vi "Main.vi"(8 "error in":errorcluster, 11 "Settings Window in":refnum<class "Settings Window.lvclass">) -> (0 "error out":errorcluster, 3 "Settings Window out":refnum<class "Settings Window.lvclass">)   [LabVIEW 2023, in "Settings Window.lvclass"]
doc: "The <b>Queued Message Handler</b> of the Worker that owns this VI."
uses:
  Settings Window.lvclass
  Settings.ctl
  Initialization Data.ctl
  Response Cases.ctl
  <vilib>/addons/_Workers/Library/Case Label.ctl
  Settings Window.lvclass/Settings Window.ctl
  rqp_Show Window.ctl
  rqp_Get Settings.ctl
  <vilib>/Utility/error.llb/Error Cluster From Error Code.vi
  <vilib>/ErrorRing/Error Ring.xnode
  <vilib>/addons/_Workers/Library/Classes/Message Queue/Message Queue.lvclass
  <vilib>/addons/_Workers/Library/Workers.lvlib
panel:
  in  "Calcs":T1 caption="Расчёты" {"B" format="%#_f"; "b" format="%#_f"; "A" format="%#_f"; "a" format="%#_f"; "K0" format="%#_f"; "Vm0" format="%#_f"}
  in  "Read Calcs":bool
  in  "Cancel Button":bool
  in  "OK Button":bool
  in  "Read Heater":bool
  in  "Heater":cluster{"P":dbl, "I":dbl} caption="Нагреватель" {"I" format="%#_f"; "P" format="%#_f"}
  in  "Read PLC2":bool
  in  "Read PLC1":bool
  in  "PLC2":cluster{"port":u16, "address":string}
  in  "PLC1":cluster{"port":u16, "address":string}
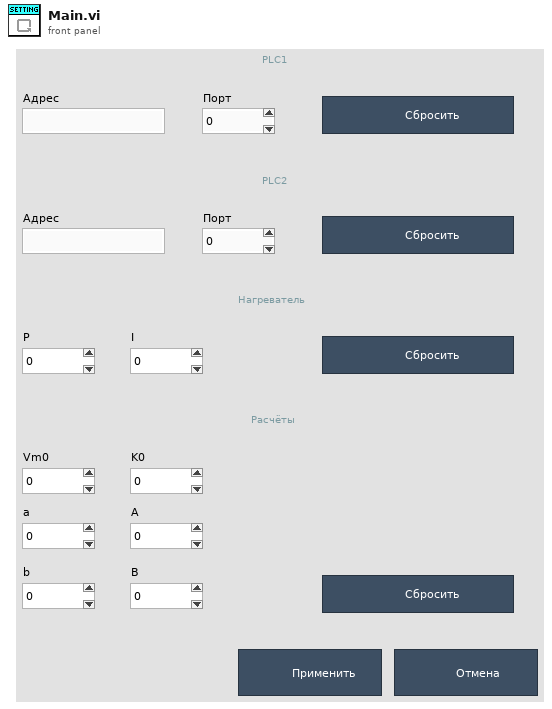
[diagram p1: front panel]
types:
  T1 = cluster{"Vm0":dbl, "K0":dbl, "a":dbl, "A":dbl, "b":dbl, "B":dbl}
  T2 = enum32{"Invalid", "Standard", "Closed", "Hidden", "Minimized", "Maximized"}
  T3 = typedef "Settings Window.lvclass/Settings.ctl" = cluster{"PLC1":cluster{"port":u16, "address":string}, "PLC2":cluster{"port":u16, "address":string}, "Heater":cluster{"P":dbl, "I":dbl}, "Calcs":cluster{"Vm0":dbl, "K0":dbl, "a_small":dbl, "A":dbl, "b_small":dbl, "B":dbl}}
  T4 = cluster{"PLC1":cluster{"port":u16, "address":string}, "PLC2":cluster{"port":u16, "address":string}, "Heater":cluster{"P":dbl, "I":dbl}, "Calcs":cluster{"Vm0":dbl, "K0":dbl, "a_small":dbl, "A":dbl, "b_small":dbl, "B":dbl}}
  T5 = typedef "Settings Window.lvclass/Initialization Data.ctl" = cluster{"Response Cases":T6, "Config Path":path}
  T6 = typedef "Settings Window.lvclass/Response Cases.ctl" = cluster{"Placeholder - Can be deleted":string, "Get Settings":T7, "Starting Settings":T7}
  T7 = typedef "Workers.lvlib/Case Label.ctl" = string
  T8 = enum16{"open", "replace", "create", "open or create", "replace or create", "replace or create with confirmation"}
  T9 = typedef "Settings Window.lvclass/rqp_Show Window.ctl" = cluster{"String":string}
  T10 = typedef "Settings Window.lvclass/rqp_Get Settings.ctl" = cluster{"String":string}
  T11 = cluster{"Vm0":dbl, "K0":dbl, "a_small":dbl, "A":dbl, "b_small":dbl, "B":dbl}
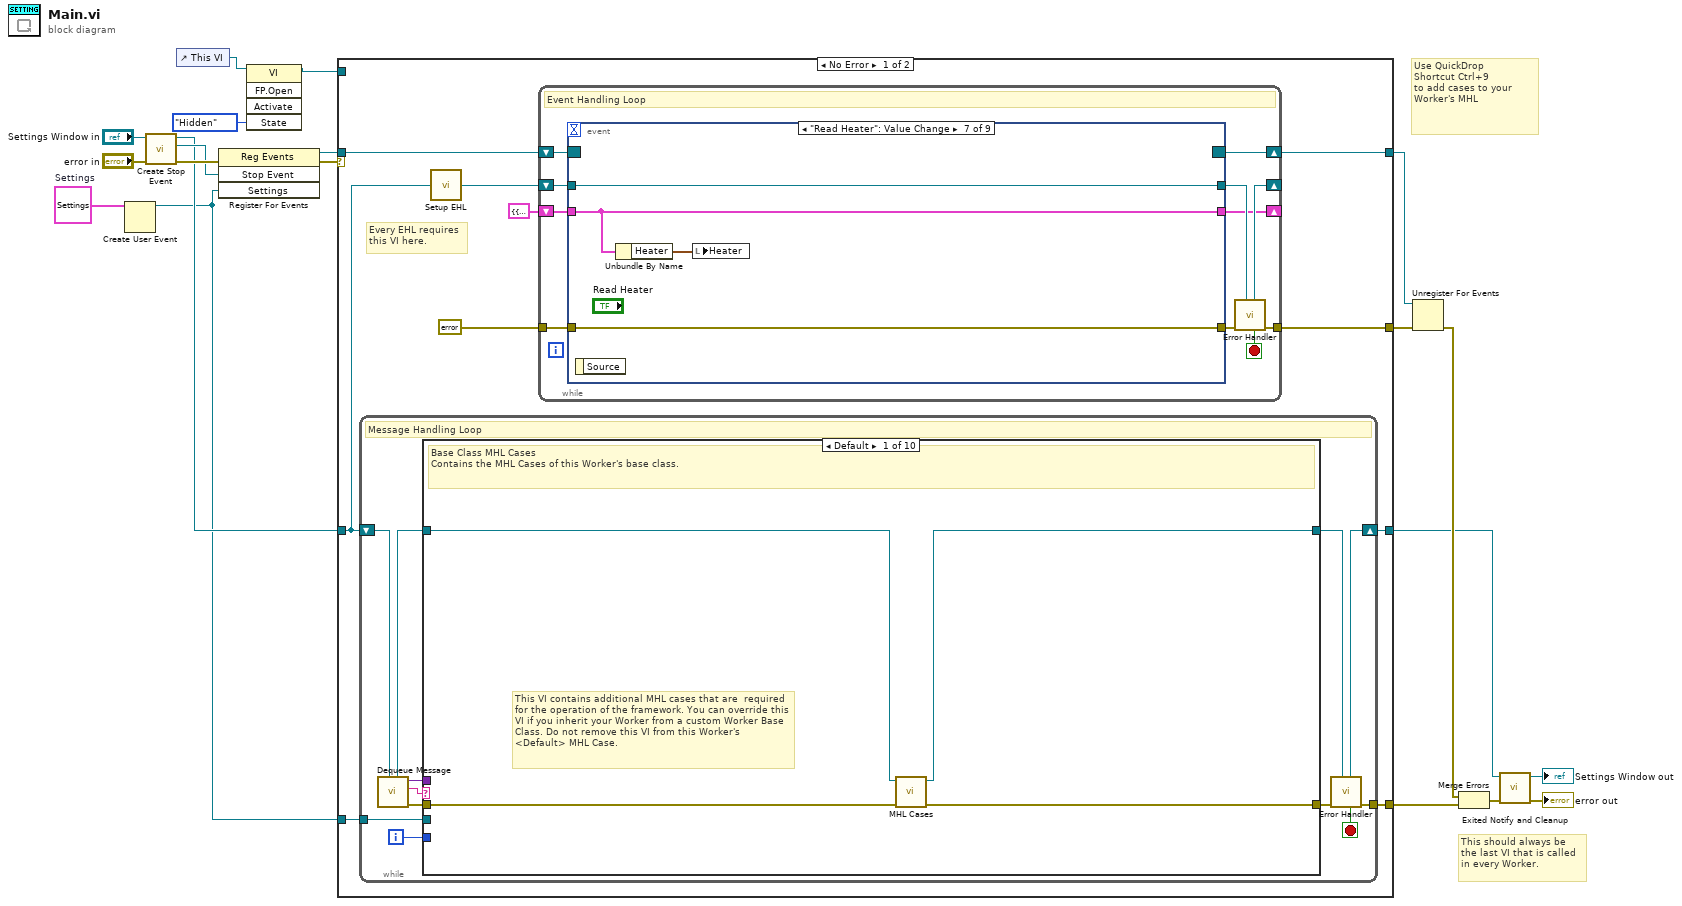
[diagram p0: block diagram]
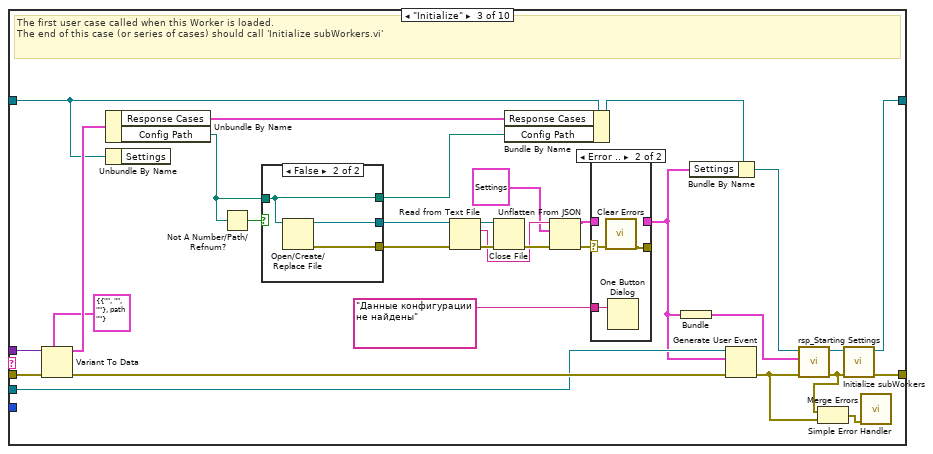
[diagram p3: hidden frame]
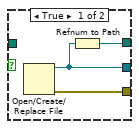
[diagram p5: hidden frame]
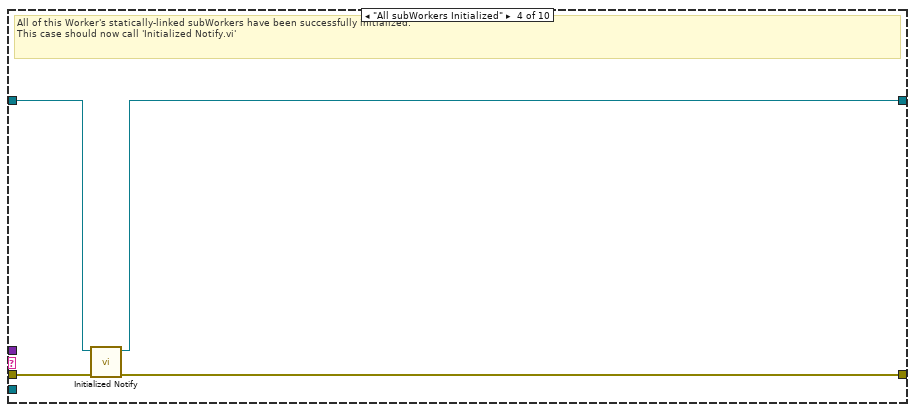
[diagram p6: hidden frame]
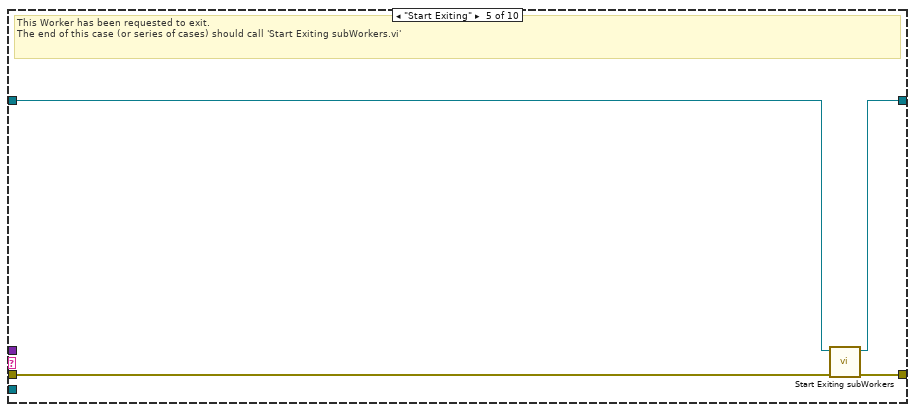
[diagram p7: hidden frame]
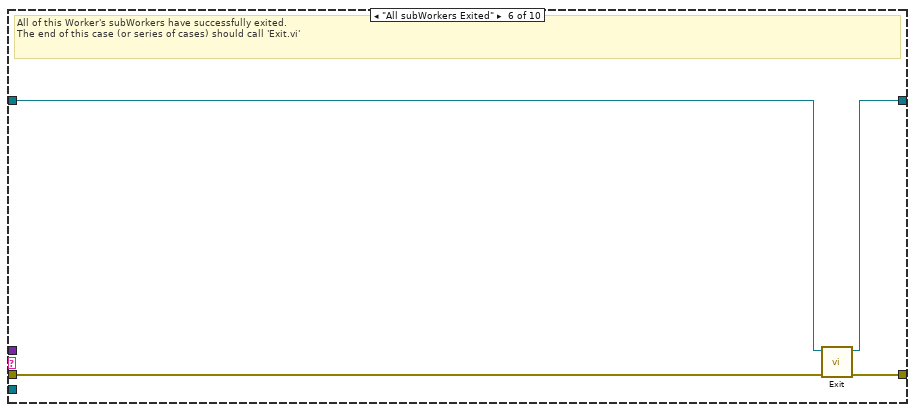
[diagram p8: hidden frame]
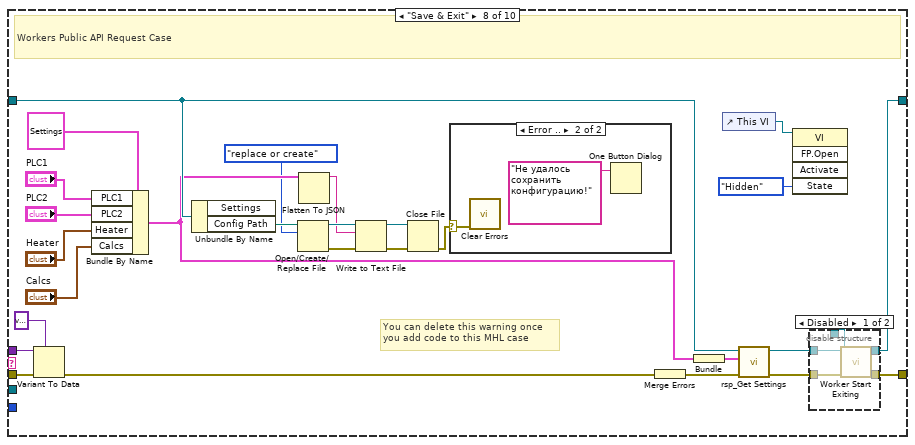
[diagram p10: hidden frame]
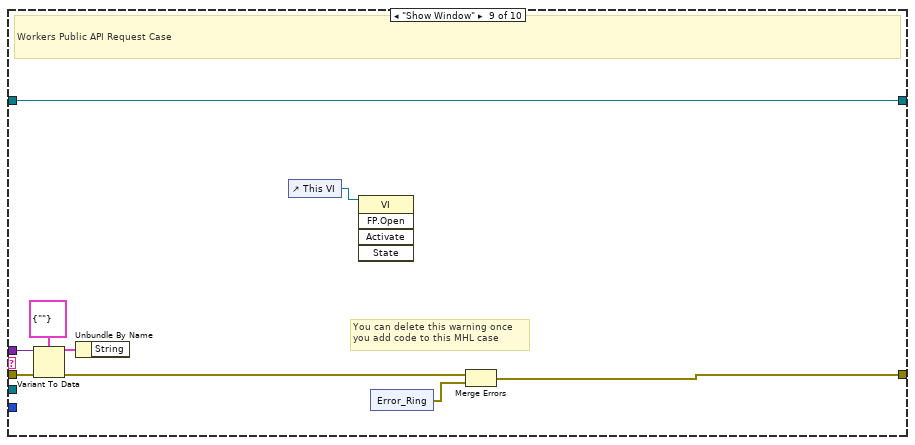
[diagram p13: hidden frame]
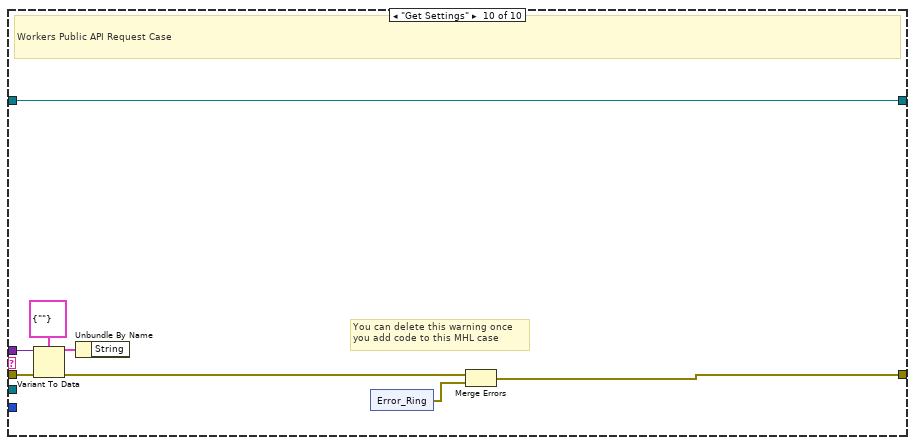
[diagram p14: hidden frame]
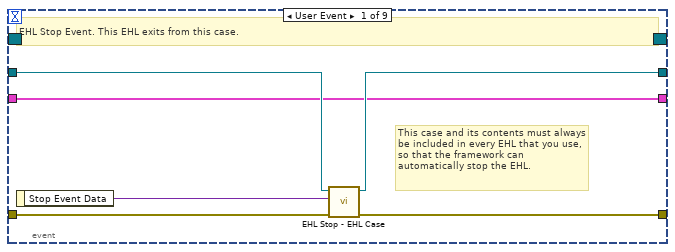
[diagram p15: hidden frame]
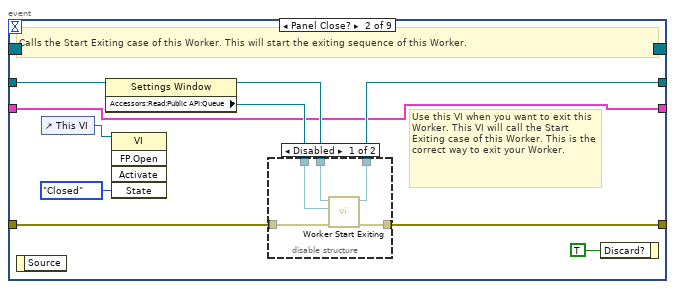
[diagram p16: hidden frame]
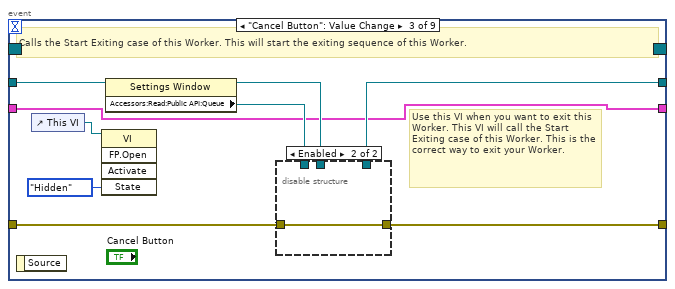
[diagram p18: hidden frame]
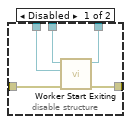
[diagram p19: hidden frame]
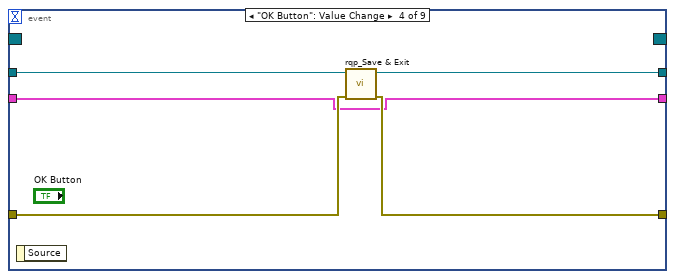
[diagram p20: hidden frame]
diagram:
  w4 = T3 {"PLC1"={"port"=0, "address"=""}, "PLC2"={"port"=0, "address"=""}, "Heater"={"P"=0.0, "I"=0.0}, "Calcs"={"Vm0"=0.0, "K0"=0.0, "a_small"=0.0, "A"=0.0, "b_small"=0.0, "B"=0.0}}  # Settings
  # "Use QuickDrop\nShortcut Ctrl+9\nto add cases to your\nWorker's MHL"
  # "This should always be the last VI that is called in every Worker."
  n1 = Create User Event(user event datatype=w4) -> (user event=w5:refnum<user-event>)  [unwired: 1 in, 1 out]
  n2 = call-dynamic "Create Stop Event.vi"("error in"="error in", "Worker"="Settings Window in") -> ("error out"=w15:errorcluster, "Stop Event"=w12:refnum<user-event>, "Worker out"=w9:refnum<class "Settings Window.lvclass">)  [unwired: 7 in]
  n3 = control-ref of="This VI"() -> (w3:refnum<vi>)
  n4 = register-events(error in=w15, w12, w5) -> (reference out=w14:refnum<event-registration>, error out=w6:errorcluster)  [unwired: 1 in]
  n5 = invoke class="VI" method="FP.Open"(reference=w3, "State"=T2."Hidden") -> (reference out=w1:refnum<vi>)  [unwired: 3 in, 4 out]
  n6 = case shown="No Error" w6 {
    tunnel: w9 -> [w22 w245]
    tunnel: [w24 w246] -> w13
    tunnel: w14 -> [w30 w247]
    tunnel: [w27 w248] -> w19
    tunnel: [w29 w247] -> w18
    tunnel: [w25 w244] -> w16
    selector: w6 -> [_ w248]
    tunnel: w5 -> [w23 _]
    tunnel: w1 -> [_ _]
    frame No Error {
      # "Every EHL requires\nthis VI here."
      n7 = while {
        shift-right: [w40] -> w25
        shift-left: w22 -> [w42]
        tunnel: [w41] -> w24
        tunnel: w23 -> [w32]
        i -> [w33]
        stop <- w34 stop-if-true
        # "Message Handling Loop"
        n8 = call-dynamic "Dequeue Message.vi"("Worker"=w42) -> ("error out"=w39:errorcluster, "Case out"=w35:string, "Data out"=w31:variant, "Worker out"=w37:refnum<class "Settings Window.lvclass">)  [unwired: 6 in, 1 out]
        n9 = case "Worker MHL Case Structure (DO NOT CHANGE LABEL NAME)" shown="Default" w35 {
          tunnel: w39 -> [w46 w47 w78 w92 w95 w102 w104 w131 w148 w161]
          tunnel: [w45 w47 w53 w91 w98 w101 w104 w117 w143 w156] -> w38
          tunnel: w37 -> [w44 w48 w68 w94 w96 w100 w103 w119 w149 w162]
          tunnel: [w43 w48 w79 w93 w97 w99 w103 w116 w149 w162] -> w36
          tunnel: w33 -> [_ _ _ _ _ _ _ _ _ _]
          tunnel: w32 -> [_ _ w61 _ _ _ _ _ _ _]
          tunnel: w31 -> [_ _ w77 _ _ _ _ w129 w145 w158]
          frame Default {
            # "This VI contains additional MHL cases that are  required for the operation of the framework. You can override this VI if you inherit your Worker from a custom Worker Base Class. Do not remove this VI from this Worker's <Default> MHL Case."
            # "Base Class MHL Cases\nContains the MHL Cases of this Worker's base class."
            n10 = call-dynamic "MHL Cases.vi"("error in"=w46, "Worker in"=w44) -> ("error out"=w45:errorcluster, "Worker out"=w43:refnum<class "Settings Window.lvclass">)  [unwired: 8 in]
          }
          frame "------------ FRAMEWORK CASES -----------" {
            # "Start of Workers Framework Cases"
          }
          frame "Initialize" {
            # "The first user case called when this Worker is loaded.\nThe end of this case (or series of cases) should call 'Initialize subWorkers.vi'"
            n11 = Variant To Data(error in=w78, type=T5 {"Response Cases"={"Placeholder - Can be deleted"="", "Get Settings"="", "Starting Settings"=""}, "Config Path"=path ""} ("Initialization Data"), Variant=w77) -> (data=w76:T5, error out=w62:errorcluster)
            n12 = Unbundle By Name(w76) -> ("Response Cases"=w75:T6, "Config Path"=w54:path)
            n13 = Unbundle By Name(w68) -> ()  [unwired: 1 out]
            n14 = Not A Number/Path/Refnum?(number/path/refnum=w54) -> (NaN/Path/Refnum?=w73:bool)
            n15 = case shown="False" w73 {
              tunnel: [w86 w90] -> w60
              tunnel: w54 -> [_ w88]
              tunnel: [w87 w89] -> w72
              tunnel: [w85 w88] -> w59
              frame True {
                n16 = Open/Create/Replace File() -> (refnum out=w86:refnum<file>, error out=w87:errorcluster)  [unwired: 6 in, 1 out]
                n17 = Refnum to Path(1:w86) -> (0:w85:path)
              }
              frame False {
                n18 = Open/Create/Replace File(file path (use dialog)=w88) -> (refnum out=w90:refnum<file>, error out=w89:errorcluster)  [unwired: 5 in, 1 out]
              }
            }
            n19 = Read from Text File(file (use dialog)=w60, error in=w72) -> (refnum out=w70:refnum<file>, text=w67:string, error out=w71:errorcluster)  [unwired: 2 in, 1 out]
            n20 = Close File(refnum=w70, error in=w71) -> (error out=w69:errorcluster)  [unwired: 1 out]
            n21 = Bundle By Name(cluster=w68, "Response Cases"=w75, "Config Path"=w59) -> (w63:refnum<class "Settings Window.lvclass">)
            n22 = Unflatten From JSON(JSON string=w67, type and defaults=T3 {"PLC1"={"port"=0, "address"=""}, "PLC2"={"port"=0, "address"=""}, "Heater"={"P"=0.0, "I"=0.0}, "Calcs"={"Vm0"=0.0, "K0"=0.0, "a_small"=0.0, "A"=0.0, "b_small"=0.0, "B"=0.0}} ("Settings"), error in (no error)=w69) -> (value=w65:T3, error out=w66:errorcluster)  [unwired: 4 in]
            n23 = case shown="Error .." w66 {
              selector: w66 -> [w80 w84]
              tunnel: [w81 _] -> w58
              tunnel: w65 -> [w81 _]
              tunnel: [w80 w83] -> _
              tunnel: "Данные конфигурации не найдены" ("message") -> [_ w82]
              frame No Error {
              }
              frame Error {
                n24 = call <vilib>:"Clear Errors.vi"("error in (no error)"=w84) -> ("error out"=w83:errorcluster)  [unwired: 5 in, 1 out]
                n25 = One Button Dialog(message=w82) -> ()  [unwired: 1 in, 1 out]
              }
            }
            n26 = Bundle("Settings"=w58) -> (w57:cluster{"Settings":T3})  [unwired: 1 in]
            n27 = Bundle By Name(cluster=w63, "Settings"=w58) -> (w56:refnum<class "Settings Window.lvclass">)
            n28 = Generate User Event(user event=w61, event data cluster=w58, error in=w62) -> (error out=w50:errorcluster)  [unwired: 1 in, 1 out]
            n29 = call "rsp_Starting Settings.vi"("error in"=w50, "Data in"=w57, "Settings Window in"=w56) -> ("error out"=w51:errorcluster, "dup Settings Window out"=w55:refnum<class "Settings Window.lvclass">)  [unwired: 7 in]
            n30 = Merge Errors(w51, w50) -> (w52:errorcluster)
            n31 = call-dynamic "Initialize subWorkers.vi"("error in"=w51, "Worker"=w55) -> ("error out"=w53:errorcluster, "dup Worker out"=w79:refnum<class "Settings Window.lvclass">)  [unwired: 8 in]
            n32 = call <vilib>:"Simple Error Handler.vi"("error in (no error)"=w52) -> ()  [unwired: 4 in, 5 out]
          }
          frame "All subWorkers Initialized" {
            # "All of this Worker's statically-linked subWorkers have been successfully initialized.\nThis case should now call 'Initialized Notify.vi'"
            n33 = call-dynamic "Initialized Notify.vi"("error in"=w92, "Worker"=w94) -> ("error out"=w91:errorcluster, "dup Worker out"=w93:refnum<class "Settings Window.lvclass">)  [unwired: 8 in]
          }
          frame "Start Exiting" {
            # "This Worker has been requested to exit. \nThe end of this case (or series of cases) should call 'Start Exiting subWorkers.vi'"
            n34 = call-dynamic "Start Exiting subWorkers.vi"("error_in"=w95, "Worker"=w96) -> ("error out"=w98:errorcluster, "dup Worker out"=w97:refnum<class "Settings Window.lvclass">)  [unwired: 8 in]
          }
          frame "All subWorkers Exited" {
            # "All of this Worker's subWorkers have successfully exited. \nThe end of this case (or series of cases) should call 'Exit.vi'"
            n35 = call-dynamic "Exit.vi"("error_in"=w102, "Worker"=w100) -> ("error out"=w101:errorcluster, "dup Worker out"=w99:refnum<class "Settings Window.lvclass">)  [unwired: 8 in]
          }
          frame "------------- PUBLIC API CASES -------------" {
            # "Start of Workers Public API Cases"
          }
          frame "Save & Exit" {
            # "You can delete this warning once\nyou add code to this MHL case"
            # "Workers Public API Request Case"
            n36 = Variant To Data(error in=w131, type=variant, Variant=w129) -> (error out=w130:errorcluster)  [unwired: 1 out]
            n37 = Bundle By Name(cluster=T3 {"PLC1"={"port"=0, "address"=""}, "PLC2"={"port"=0, "address"=""}, "Heater"={"P"=0.0, "I"=0.0}, "Calcs"={"Vm0"=0.0, "K0"=0.0, "a_small"=0.0, "A"=0.0, "b_small"=0.0, "B"=0.0}} ("Settings"), "PLC1"="PLC1", "PLC2"="PLC2", "Heater"="Heater", "Calcs"="Calcs") -> (w111:T3)
            n38 = Unbundle By Name(w119) -> ("Config Path"=w128:path)  [unwired: 1 out]
            n39 = Open/Create/Replace File(file path (use dialog)=w128, operation (0:open)=T8."replace or create") -> (refnum out=w126:refnum<file>, error out=w127:errorcluster)  [unwired: 4 in, 1 out]
            n40 = Flatten To JSON(anything=w111) -> (JSON string=w122:string)  [unwired: 2 in, 1 out]
            n41 = Write to Text File(file (use dialog)=w126, text=w122, error in=w127) -> (refnum out=w120:refnum<file>, error out=w121:errorcluster)  [unwired: 1 in, 1 out]
            n42 = Close File(refnum=w120, error in=w121) -> (error out=w114:errorcluster)  [unwired: 1 out]
            n43 = case shown="Error .." w114 {
              selector: w114 -> [_ w139]
              frame No Error {
              }
              frame Error {
                n44 = call <vilib>:"Clear Errors.vi"("error in (no error)"=w139) -> ()  [unwired: 5 in, 2 out]
                n45 = One Button Dialog(message="Не удалось сохранить конфигурацию!") -> ()  [unwired: 1 in, 1 out]
              }
            }
            n46 = Merge Errors(w130) -> (w118:errorcluster)
            n47 = Bundle("Settings"=w111) -> (w109:cluster{"Settings":T3})  [unwired: 1 in]
            n48 = control-ref of="This VI"() -> (w107:refnum<vi>)
            n49 = call "rsp_Get Settings.vi"("error in"=w118, "Data in"=w109, "Settings Window in"=w119) -> ("error out"=w112:errorcluster, "dup Settings Window out"=w113:refnum<class "Settings Window.lvclass">)  [unwired: 7 in]
            n50 = invoke class="VI" method="FP.Open"(reference=w107, "State"=T2."Hidden") -> ()  [unwired: 3 in, 5 out]
            n51 = disable-structure shown="Disabled" {
              disable-tunnel: [w136 w137] -> w117
              disable-tunnel: _ -> [w135 _]
              disable-tunnel: [w134 w138] -> w116
              disable-tunnel: w113 -> [w133 w138]
              disable-tunnel: w112 -> [w132 w137]
              frame Disabled {
                n52 = call-dynamic "Worker Start Exiting.vi"("error_in"=w132, "Message Queue"=w135, "Worker"=w133) -> ("error out"=w136:errorcluster, "dup Worker out"=w134:refnum<class "Settings Window.lvclass">)  [unwired: 7 in]
              }
              frame Enabled {
              }
            }
          }
          frame "Show Window" {
            # "You can delete this warning once\nyou add code to this MHL case"
            # "Workers Public API Request Case"
            n53 = Variant To Data(error in=w148, type=T9 {"String"=""} ("Data"), Variant=w145) -> (data=w144:T9, error out=w147:errorcluster)
            n54 = Unbundle By Name(w144) -> ()  [unwired: 1 out]
            n55 = control-ref of="This VI"() -> (w141:refnum<vi>)
            n56 = invoke class="VI" method="FP.Open"(reference=w141) -> ()  [unwired: 4 in, 5 out]
            n57 = xnode ("Error_Ring")() -> ("error out"=w142:errorcluster)
            n58 = Merge Errors(w147, w142) -> (w143:errorcluster)
          }
          frame "Get Settings" {
            # "You can delete this warning once\nyou add code to this MHL case"
            # "Workers Public API Request Case"
            n59 = Variant To Data(error in=w161, type=T10 {"String"=""} ("Data"), Variant=w158) -> (data=w157:T10, error out=w160:errorcluster)
            n60 = Unbundle By Name(w157) -> ()  [unwired: 1 out]
            n61 = xnode ("Error_Ring")() -> ("error out"=w155:errorcluster)
            n62 = Merge Errors(w160, w155) -> (w156:errorcluster)
          }
        }
        n63 = call-dynamic "Error Handler.vi"("Worker"=w36, "error_in"=w38) -> ("error out"=w41:errorcluster, "Stop Loop"=w34:bool, "Worker out"=w40:refnum<class "Settings Window.lvclass">)  [unwired: 7 in]
      }
      n64 = call-dynamic "Setup EHL.vi"("Worker"=w22) -> ("Worker out"=w26:refnum<class "Settings Window.lvclass">)  [unwired: 14 in]
      n65 = while "Event Handling Loop" {
        shift-right: [w178] -> w29
        shift-left: w30 -> [w177]
        tunnel: [w173] -> w27
        tunnel: errorcluster {"status"=FALSE, "code"=0, "source"=""} ("error constant") -> [w175]
        shift-right: [w171] -> _
        shift-left: w26 -> [w176]
        shift-right: [w169] -> _
        shift-left: T4 {"PLC1"={"port"=0, "address"=""}, "PLC2"={"port"=0, "address"=""}, "Heater"={"P"=0.0, "I"=0.0}, "Calcs"={"Vm0"=0.0, "K0"=0.0, "a_small"=0.0, "A"=0.0, "b_small"=0.0, "B"=0.0}} -> [w168]
        stop <- w170 stop-if-true
        # "Event Handling Loop"
        n66 = event shown="[6] \"Read Heater\": Value Change" {
          selector: w177 -> [_ _ _ _ _ _ _ _ _]
          dyn-events: [_ _ _ _ _ _ _ _ _] -> w178
          timeout: _ -> [_ _ _ _ _ _ _ _ _]
          tunnel: [w183 w193 w209 w217 w224 w228 w232 w236 w243] -> w174
          tunnel: w175 -> [w184 w192 w208 w218 w224 w228 w232 w236 w243]
          tunnel: w176 -> [w182 w191 w207 w220 w223 w227 w231 w235 w242]
          tunnel: [w181 w190 w206 w219 w223 w227 w231 w235 w242] -> w172
          tunnel: [w179 w185 w201 w216 w222 w226 w230 w234 w237] -> w169
          tunnel: w168 -> [w179 w185 w201 w216 w222 w226 w230 w234 _]
          event User Event {
            # "This case and its contents must always be included in every EHL that you use, so that the framework can automatically stop the EHL."
            # "EHL Stop Event. This EHL exits from this case."
            n67 = event-data() -> ("Stop Event Data"=w180:variant)  [unwired: 1 in]
            n68 = call-dynamic "EHL Stop - EHL Case.vi"("error in"=w184, "Stop Event Data"=w180, "Worker"=w182) -> ("error out"=w183:errorcluster, "Worker out"=w181:refnum<class "Settings Window.lvclass">)  [unwired: 7 in]
          }
          event Panel Close? {
            # "Use this VI when you want to exit this Worker. This VI will call the Start Exiting case of this Worker. This is the correct way to exit your Worker."
            # "Calls the Start Exiting case of this Worker. This will start the exiting sequence of this Worker."
            n69 = event-data() -> ()  [unwired: 1 in, 1 out]
            n70 = control-ref of="This VI"() -> (w187:refnum<vi>)
            n71 = property class="Settings Window"(reference=w191) -> (reference out=w189:refnum<class "Settings Window.lvclass">, "Accessors:Read:Public API:Queue"=w188:refnum<class "Message Queue.lvclass">)  [unwired: 1 in, 1 out]
            n72 = invoke class="VI" method="FP.Open"(reference=w187, "State"=T2."Closed") -> ()  [unwired: 3 in, 5 out]
            n73 = disable-structure shown="Disabled" {
              disable-tunnel: [w199 w200] -> w193
              disable-tunnel: w192 -> [w198 w200]
              disable-tunnel: [w197 _] -> w190
              disable-tunnel: w189 -> [w196 _]
              disable-tunnel: w188 -> [w195 _]
              frame Disabled {
                n74 = call-dynamic "Worker Start Exiting.vi"("error_in"=w198, "Message Queue"=w195, "Worker"=w196) -> ("error out"=w199:errorcluster, "dup Worker out"=w197:refnum<class "Settings Window.lvclass">)  [unwired: 7 in]
              }
              frame Enabled {
              }
            }
            n75 = event-data("Discard?"=TRUE) -> ()  [unwired: 1 in, 1 out]
          }
          event "Cancel Button": Value Change {
            # "Use this VI when you want to exit this Worker. This VI will call the Start Exiting case of this Worker. This is the correct way to exit your Worker."
            # "Calls the Start Exiting case of this Worker. This will start the exiting sequence of this Worker."
            n76 = event-data() -> ()  [unwired: 1 in, 1 out]
            n77 = control-ref of="This VI"() -> (w203:refnum<vi>)
            n78 = invoke class="VI" method="FP.Open"(reference=w203, "State"=T2."Hidden") -> ()  [unwired: 3 in, 5 out]
            n79 = property class="Settings Window"(reference=w207) -> (reference out=w205:refnum<class "Settings Window.lvclass">, "Accessors:Read:Public API:Queue"=w204:refnum<class "Message Queue.lvclass">)  [unwired: 1 in, 1 out]
            n80 = disable-structure shown="Enabled" {
              disable-tunnel: [w214 w215] -> w209
              disable-tunnel: w208 -> [w213 w215]
              disable-tunnel: [w212 _] -> w206
              disable-tunnel: w205 -> [w211 _]
              disable-tunnel: w204 -> [w210 _]
              frame Disabled {
                n81 = call-dynamic "Worker Start Exiting.vi"("error_in"=w213, "Message Queue"=w210, "Worker"=w211) -> ("error out"=w214:errorcluster, "dup Worker out"=w212:refnum<class "Settings Window.lvclass">)  [unwired: 7 in]
              }
              frame Enabled {
              }
            }
          }
          event "OK Button": Value Change {
            n82 = event-data() -> ()  [unwired: 1 in, 1 out]
            n83 = call "rqp_Save & Exit.vi"("error in"=w218, "Settings Window in"=w220) -> ("error out"=w217:errorcluster, "dup Settings Window out"=w219:refnum<class "Settings Window.lvclass">)  [unwired: 7 in, 1 out]
          }
          event "Read PLC1": Value Change {
            n84 = event-data() -> ()  [unwired: 1 in, 1 out]
            n85 = Unbundle By Name(w222) -> ("PLC1"=w221:cluster{"port":u16, "address":string})
            n86 = local write "PLC1"(w221) -> ()
          }
          event "Read PLC2": Value Change {
            n87 = event-data() -> ()  [unwired: 1 in, 1 out]
            n88 = Unbundle By Name(w226) -> ("PLC2"=w225:cluster{"port":u16, "address":string})
            n89 = local write "PLC2"(w225) -> ()
          }
          event "Read Heater": Value Change {
            n90 = event-data() -> ()  [unwired: 1 in, 1 out]
            n91 = Unbundle By Name(w230) -> ("Heater"=w229:cluster{"P":dbl, "I":dbl})
            n92 = local write "Heater"(w229) -> ()
          }
          event "Read Calcs": Value Change {
            n93 = event-data() -> ()  [unwired: 1 in, 1 out]
            n94 = Unbundle By Name(w234) -> ("Calcs"=w233:T11)
            n95 = local write "Calcs"(w233) -> ()
          }
          event User Event {
            n96 = event-data() -> ("PLC1"=w241:cluster{"port":u16, "address":string}, "PLC2"=w240:cluster{"port":u16, "address":string}, "Heater"=w239:cluster{"P":dbl, "I":dbl}, "Calcs"=w238:T11)  [unwired: 1 in]
            n97 = Bundle("PLC1"=w241, "PLC2"=w240, "Heater"=w239, "Calcs"=w238) -> (w237:T4)  [unwired: 1 in]
            n98 = local write "PLC1"(w241) -> ()
            n99 = local write "PLC2"(w240) -> ()
            n100 = local write "Heater"(w239) -> ()
            n101 = local write "Calcs"(w238) -> ()
          }
        }
        n102 = call-dynamic "Error Handler.vi"("Worker"=w172, "error_in"=w174) -> ("error out"=w173:errorcluster, "Stop Loop"=w170:bool, "Worker out"=w171:refnum<class "Settings Window.lvclass">)  [unwired: 7 in]
      }
    }
    frame Error {
      n103 = call-dynamic "Error Handler.vi"("Worker"=w245, "error_in"=w248) -> ("error out"=w246:errorcluster, "Worker out"=w244:refnum<class "Settings Window.lvclass">)  [unwired: 7 in, 1 out]
    }
  }
  n104 = Unregister For Events(event registration refnum=w18, error in=w19) -> (error out=w20:errorcluster)
  n105 = Merge Errors(w20, w13) -> (w17:errorcluster)
  n106 = call-dynamic "Exited Notify and Cleanup.vi"("error_in"=w17, "Worker"=w16) -> ("error out"=→"error out":errorcluster, "dup Worker out"=→"Settings Window out":refnum<class "Settings Window.lvclass">)  [unwired: 8 in]
